vi "TCP - Asynchronous Write.vi"(8 "error in":errorcluster, 10 "Message to Send":string, 11 "TCP Network Connection in":refnum<k5>) -> (0 "error out":errorcluster, 3 "TCP Network Connection out":refnum<k5>)   [LabVIEW 2021]
doc: "Send an asynchronous message through TCP"
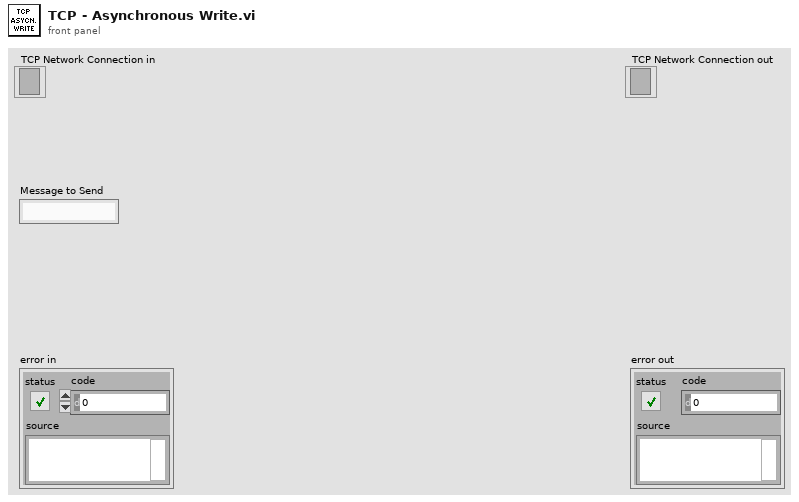
[diagram p1: front panel]
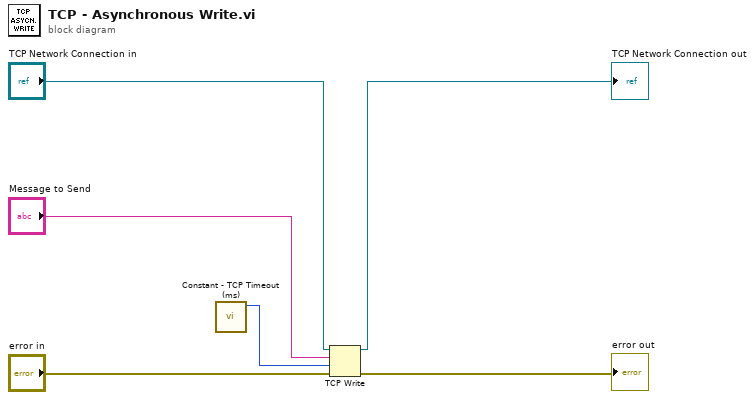
[diagram p0: block diagram]
diagram:
  n1 = call "Constant - TCP Timeout (ms).vi"() -> ("timeout (ms)"=w1:i32)  [unwired: 11 in]
  n2 = TCP Write(connection ID="TCP Network Connection in", data in="Message to Send", error in (no error)="error in", 9:w1) -> (connection ID out=→"TCP Network Connection out":refnum<k5>, error out=→"error out":errorcluster)  [unwired: 1 out]
